vi "Time to Samples.vi"(7 "Time":dbl, 12 "Sample Rate":dbl) -> (8 "Samples":u32)   [LabVIEW 2016, in "SG.lvlib"]
uses:
  SG.lvlib
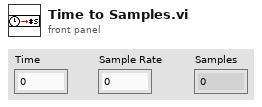
[diagram p1: front panel]
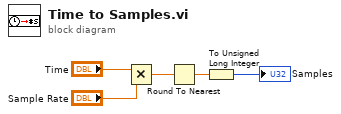
[diagram p0: block diagram]
diagram:
  n1 = Multiply(x="Time", y="Sample Rate") -> (x*y=w3:dbl)
  n2 = Round To Nearest(number=w3) -> (nearest integer value=w2:dbl)
  n3 = To Unsigned Long Integer(number=w2) -> (unsigned 32bit integer=→"Samples":u32)
